vi "DoE_Create_Standalone.vi"(11 "Input DoE Values":string[][](table)) -> (1 "written file already exists (and overwritten)":bool caption="exists", 3 "file write cancelled":bool caption="cancelled")   [LabVIEW 2015]
uses:
  <vilib>/Utility/file.llb/Write To Spreadsheet File (DBL).vi
panel:
  # "DoE_Create.vi"
  # "Pump 1"
  # "Pump 2"
  # "Pump 3"
  # "Pump 4"
  # "Temp"
  # "Run Time"
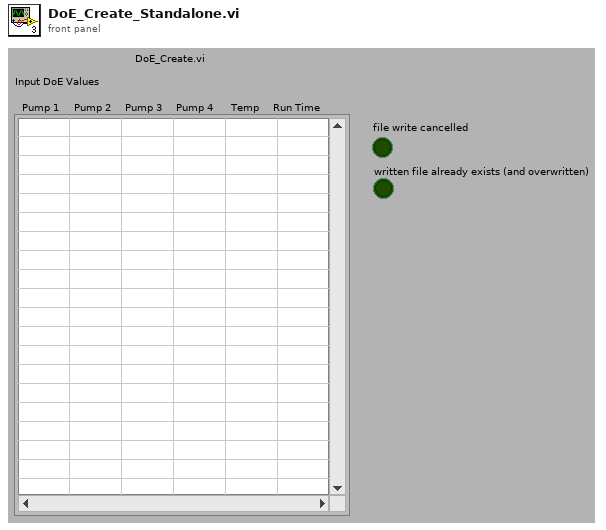
[diagram p1: front panel]
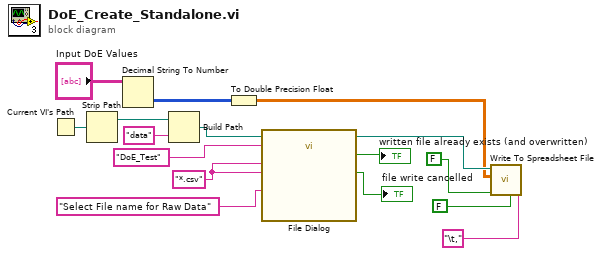
[diagram p0: block diagram]
diagram:
  w3 = "*.csv" ("pattern (all files)")
  n1 = Current VI's Path() -> (path=w13:path)
  n2 = Strip Path(path=w13) -> (stripped path=w14:path)  [unwired: 1 out]
  n3 = Decimal String To Number(string="Input DoE Values") -> (number=w16:i32[][])  [unwired: 2 in, 1 out]
  n4 = Build Path(base path=w14, name or relative path="data") -> (appended path=w11:path)
  n5 = To Double Precision Float(number=w16) -> (double precision float=w1:dbl[][])
  n6 = call "File Dialog"("start path"=w11, "prompt"="Select File name for Raw Data", "default name"="DoE_Test", "pattern (all files)"=w3, "pattern label"=w3) -> ("selected path"=w7:path, "exists"=→"written file already exists (and overwritten)":bool, "cancelled"=→"file write cancelled":bool)  [unwired: 7 in, 1 out]
  n7 = call-poly <vilib>:"Write To Spreadsheet File.vi"("delimiter (\\t)"="\t," ("delimiter (\\t)"), "transpose? (no:F)"=FALSE, "append to file? (new file:F)"=FALSE, "2D data"=w1, "file path (dialog if empty)"=w7) -> ()  [unwired: 3 in, 1 out]
